vi "Endpoint-Edit Configuration.vi"(11 "Endpoint Config In":T3[](array[typedef])) -> (3 "Endpoint Config Out":T3[](array[typedef]))   [LabVIEW 2020]
uses:
  LV Source/Endpoint-Spec.ctl
  LV Source/Endpoint-Modality.ctl
  LV Source/Endpoint-Laterality.ctl
  D:/Experiment VIs/Calibration VIs/Endpoint VIs/dotNET Source/EndpointConfigControls/bin/Release/EndpointConfigControls.dll
  dotNET Source/EndpointConfigControls/bin/Release/EndpointConfigControls.dll
panel:
  in  "Remove Button":bool
  in  "Add Button":bool
  in  "Laterality":T1
  in  "Modality":T2
  out "exit signal":bool
  in  "EndpointTable":refnum<k24>(container)
  in  "Cancel Button":bool
  in  "OK Button":bool
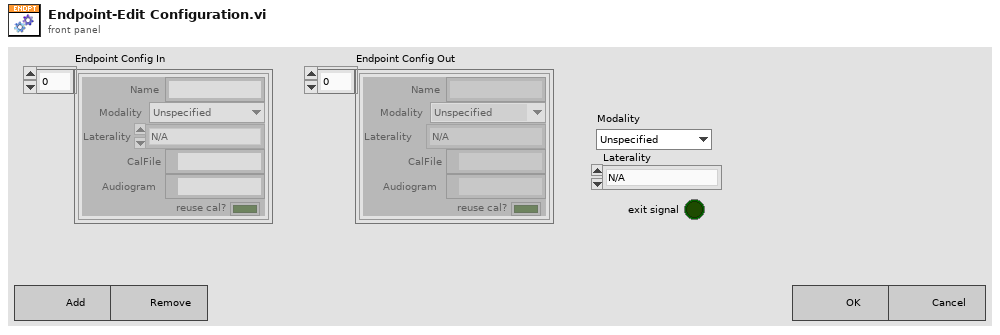
[diagram p1: front panel]
types:
  T1 = typedef "Endpoint-Laterality.ctl" = enum16{"N/A", "Right", "Left"}
  T2 = typedef "Endpoint-Modality.ctl" = enum16{"Unspecified", "Acoustic", "Electric", "Optical"}
  T3 = typedef "Endpoint-Spec.ctl" = cluster{"Name":string, "Modality":T2, "Laterality":T1, "CalFile":path, "Audiogram":path, "reuse cal?":bool}
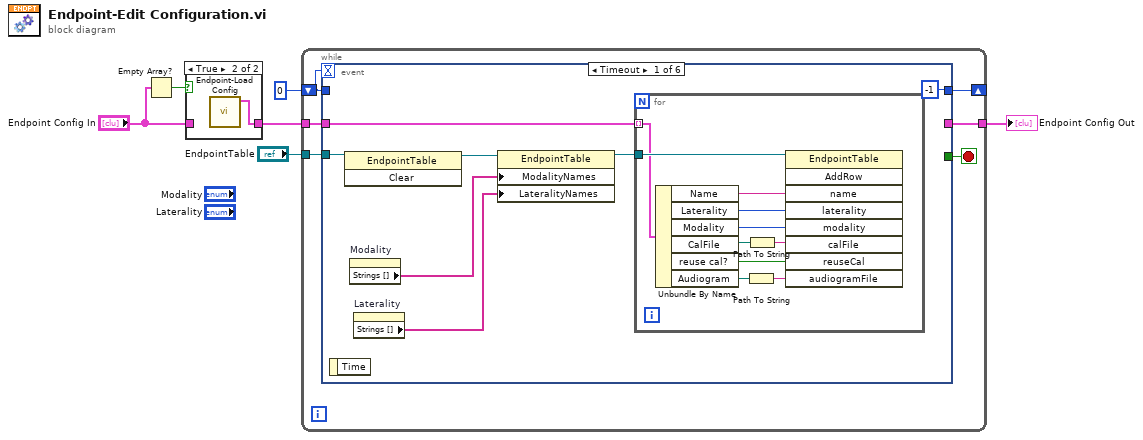
[diagram p0: block diagram]
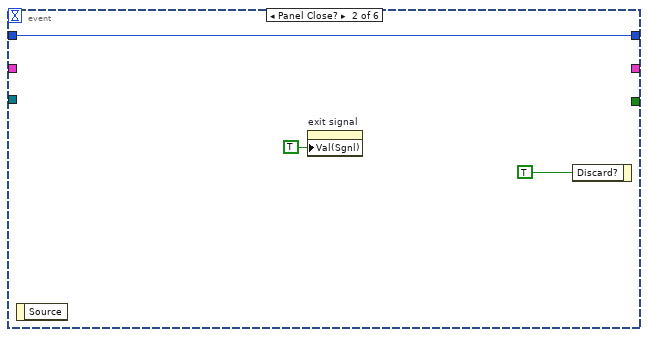
[diagram p3: hidden frame]
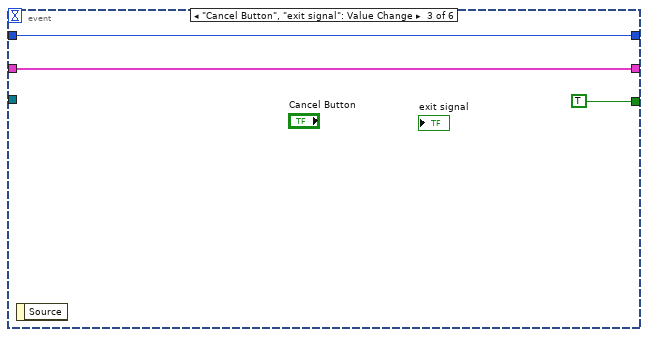
[diagram p4: hidden frame]
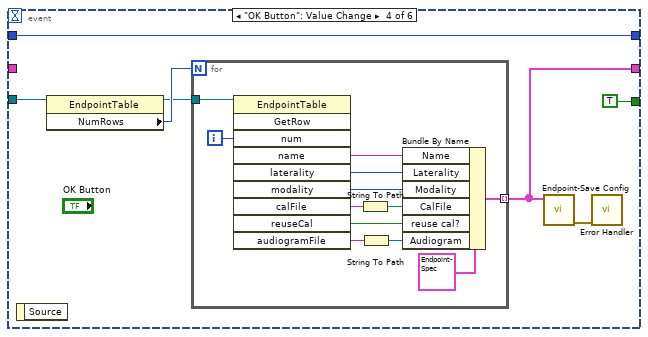
[diagram p5: hidden frame]
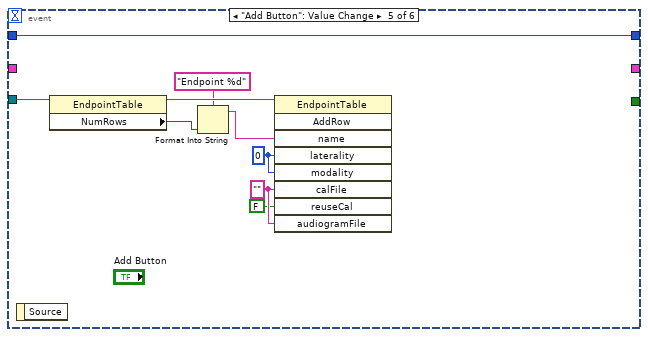
[diagram p6: hidden frame]
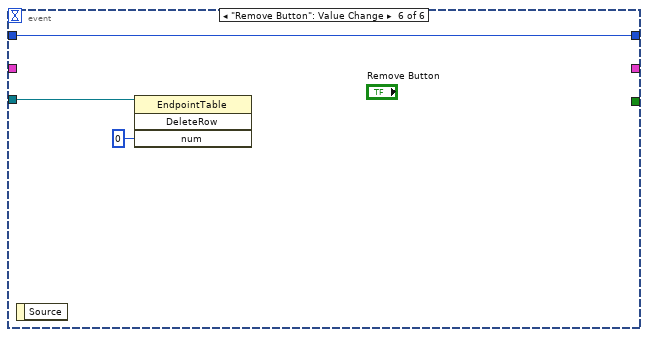
[diagram p7: hidden frame]
diagram:
  n1 = Empty Array?(array="Endpoint Config In") -> (empty?=w3:bool)
  n2 = case shown="True" w3 {
    tunnel: [w7 w8] -> w2
    tunnel: "Endpoint Config In" -> [w7 _]
    frame False {
    }
    frame True {
      n3 = call "Endpoint-Load Config.vi"() -> ("Endpoint Config"=w8:T3[])  [unwired: 10 in, 1 out]
    }
  }
  n4 = while {
    shift-right: [w13] -> _
    shift-left: 0 -> [w14]
    tunnel: [w12] -> w5
    tunnel: w2 -> [w11]
    tunnel: "EndpointTable" -> [w10]
    stop <- w9 stop-if-true
    n5 = event shown="[0] Timeout" {
      selector: _ -> [_ _ _ _ _ _]
      dyn-events: _ -> [_ _ _ _ _ _]
      timeout: w14 -> [_ _ _ _ _ _]
      tunnel: w14 -> [_ w34 w37 w44 w65 w68]
      tunnel: [-1 w34 w37 w44 w65 w68] -> w13
      tunnel: [_ _ w36 w40 _ _] -> w12
      tunnel: w11 -> [w17 _ w36 _ _ _]
      tunnel: w10 -> [w16 _ _ w43 w64 w67]
      tunnel: [_ _ TRUE TRUE _ _] -> w9
      event Timeout {
        n6 = event-data() -> ()  [unwired: 1 in, 1 out]
        n7 = invoke class="EndpointTable" method="Clear"(reference=w16) -> (reference out=w15:refnum<k24>)  [unwired: 2 in, 2 out]
        n8 = property on="Modality" class="Enum (strict)"() -> ("Strings []"=w20:string[])  [unwired: 2 in, 2 out]
        n9 = property on="Laterality" class="Enum (strict)"() -> ("Strings []"=w19:string[])  [unwired: 2 in, 2 out]
        n10 = property class="EndpointTable"(reference=w15, "ModalityNames"=w20, "LateralityNames"=w19) -> (reference out=w18:refnum<k24>)  [unwired: 1 in, 1 out]
        n11 = for {
          tunnel: w18 -> [w31]
          tunnel: w17 -> [w30] mode=indexing
          n12 = Unbundle By Name(w30) -> ("Name"=w29:string, "Laterality"=w28:T1, "Modality"=w27:T2, "CalFile"=w26:path, "reuse cal?"=w24:bool, "Audiogram"=w23:path)
          n13 = Path To String(path=w23) -> (string=w22:string)
          n14 = Path To String(path=w26) -> (string=w25:string)
          n15 = invoke class="EndpointTable" method="AddRow"(reference=w31, "name"=w29, "laterality"=w28, "modality"=w27, "calFile"=w25, "reuseCal"=w24, "audiogramFile"=w22) -> ()  [unwired: 2 in, 9 out]
        }
      }
      event Panel Close? {
        n16 = event-data() -> ()  [unwired: 1 in, 1 out]
        n17 = property on="exit signal" class="Bool (strict)"("Val(Sgnl)"=TRUE ("Value (Signaling)")) -> ()  [unwired: 2 in, 2 out]
        n18 = event-data("Discard?"=TRUE) -> ()  [unwired: 1 in, 1 out]
      }
      event "Cancel Button", "exit signal": Value Change {
        n19 = event-data() -> ()  [unwired: 1 in, 1 out]
      }
      event "OK Button": Value Change {
        n20 = event-data() -> ()  [unwired: 1 in, 1 out]
        n21 = property class="EndpointTable"(reference=w43) -> (reference out=w41:refnum<k24>, "NumRows"=w42:i32)  [unwired: 1 in, 1 out]
        n22 = for {
          N: w42 -> [_]
          tunnel: w41 -> [w56]
          tunnel: [w45] -> w40 mode=indexing
          i -> [w54]
          n23 = invoke class="EndpointTable" method="GetRow"(reference=w56, "num"=w54) -> ("name"=w53:string, "laterality"=w52:i32, "modality"=w51:i32, "calFile"=w50:string, "reuseCal"=w48:bool, "audiogramFile"=w47:string)  [unwired: 8 in, 4 out]
          n24 = String To Path(string=w50) -> (path=w49:path)
          n25 = String To Path(string=w47) -> (path=w46:path)
          n26 = Bundle By Name(cluster=T3 {"Name"="", "Modality"=enum."Unspecified", "Laterality"=enum."N/A", "CalFile"=path "", "Audiogram"=path "", "reuse cal?"=FALSE} ("Endpoint Spec"), "Name"=w53, "Laterality"=w52, "Modality"=w51, "CalFile"=w49, "reuse cal?"=w48, "Audiogram"=w46) -> (w45:T3)
        }
        n27 = call "Endpoint-Save Config.vi"("Endpoint Config"=w40) -> ("Error Out"=w39:errorcluster)  [unwired: 10 in]
        n28 = call "Error Handler.vi"("error in (no error)"=w39) -> ()  [unwired: 13 in, 2 out]
      }
      event "Add Button": Value Change {
        w58 = "" ("calFile")
        w59 = 0 ("laterality")
        n29 = event-data() -> ()  [unwired: 1 in, 1 out]
        n30 = property class="EndpointTable"(reference=w64) -> (reference out=w63:refnum<k24>, "NumRows"=w62:i32)  [unwired: 1 in, 1 out]
        n31 = Format Into String(format string="Endpoint %d", w62) -> (resulting string=w60:string)  [unwired: 2 in, 1 out]
        n32 = invoke class="EndpointTable" method="AddRow"(reference=w63, "name"=w60, "laterality"=w59, "modality"=w59, "calFile"=w58, "reuseCal"=FALSE, "audiogramFile"=w58) -> ()  [unwired: 2 in, 9 out]
      }
      event "Remove Button": Value Change {
        n33 = event-data() -> ()  [unwired: 1 in, 1 out]
        n34 = invoke class="EndpointTable" method="DeleteRow"(reference=w67, "num"=0) -> ()  [unwired: 2 in, 4 out]
      }
    }
  }
  "Endpoint Config Out" <- w5
